vi "CPAR.vi"(8 "error in (no error)":errorcluster, 10 "Parameter":string, 11 "connection ID":refnum<k16>) -> (0 "error out":errorcluster, 2 "data out":string, 3 "connection ID out":refnum<k16>)   [LabVIEW 2018]
panel:
  in  "port or service name":u16=2047
  in  "name":string="192.168.1.12"
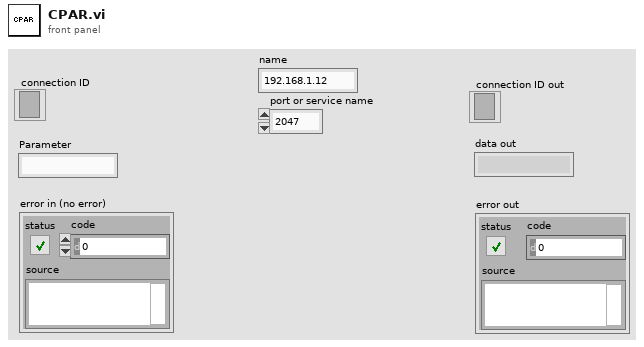
[diagram p1: front panel]
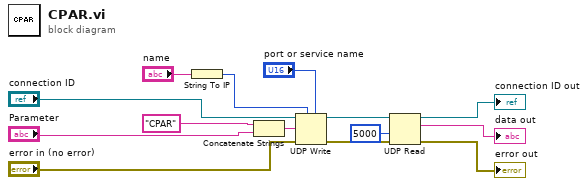
[diagram p0: block diagram]
diagram:
  n1 = String To IP(1:"name") -> (0:w9:u32)
  n2 = Concatenate Strings("CPAR" ("data in"), "Parameter") -> (w13:string)
  n3 = UDP Write(address=w9, port or service name="port or service name", connection ID="connection ID", data in=w13, 8:"error in (no error)") -> (error out=w11:errorcluster, 3:w10:refnum<k16>)  [unwired: 1 in]
  n4 = UDP Read(connection ID=w10, timeout ms (25000)=5000, 8:w11) -> (data out=→"data out":string, error out=→"error out":errorcluster, 3:→"connection ID out":refnum<k16>)  [unwired: 1 in, 2 out]
